vi "ZPL Read Set Current.vi"(6 "Settle (1 mS)":u32=1, 8 "error":errorcluster, 11 "VISA":refnum<visa-resource-name>) -> (0 "error out":errorcluster, 2 "Read Set Current":dbl format="%.4f", 3 "VISA out":refnum<visa-resource-name>)   [LabVIEW 2016]
doc: "This VI returns the current limit setting. These settings may not be the same as the actual output current."
panel:
  # "Lambda ZPLUS \n Serial Port\n  DC Power Supplies"
  # "Read the\nSet Current"
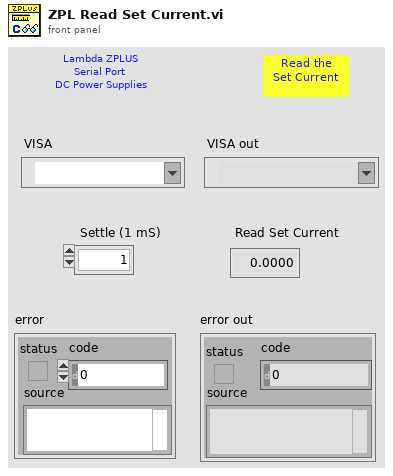
[diagram p1: front panel]
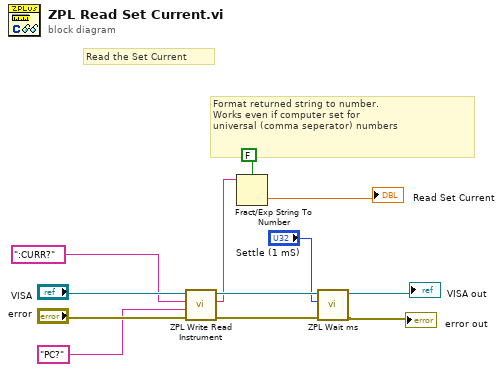
[diagram p0: block diagram]
diagram:
  # "Format returned string to number.\nWorks even if computer set for \nuniversal (comma seperator) numbers"
  # "Read the Set Current"
  n1 = call "ZPL Write Read Instrument.vi"("error in"="error", "Write Command/Query GEN"="PC?" ("format string"), "Write Command/Query SCPI"=":CURR?" ("format string"), "VISA"="VISA") -> ("error out"=w9:errorcluster, "Response"=w1:string, "VISA  out"=w10:refnum<visa-resource-name>)  [unwired: 5 in]
  n2 = Fract/Exp String To Number(use system decimal point (T)=FALSE, string=w1) -> (number=→"Read Set Current":dbl)  [unwired: 2 in, 1 out]
  n3 = call "ZPL Wait ms.vi"("error"=w9, "Delay (1 mS)"="Settle (1 mS)", "VISA"=w10) -> ("error out"=→"error out":errorcluster, "VISA out"=→"VISA out":refnum<visa-resource-name>)  [unwired: 7 in]
